vi "SerialASCII.vi"(11 "SerialASCIISettings":T1={"SerialPort"="RS232\\Port1", "TxFIFO"="DLRS1ADisplacementTxFIFO", "RxFIFO"="DLRS1ADisplacementRxFIFO", "TimestampRegister"="TimestampRegister", "Terminator"=10, "ReadTimeoutMs"=500}) -> ()   [LabVIEW 2016, in "FPGASerialASCII.lvlib"]
uses:
  FPGASerialASCII.lvlib
  DataTypes/SerialASCIISettings.ctl
  <vilib>/rvi/Emulation/niFpgaGetClockAttributes.vi
  <vilib>/rvi/Emulation/niFpgaSctlEmulationGetInTimedLoop.vi
  <vilib>/rvi/Emulation/niFpgaEmulationReportErrorSimple.vi
  <vilib>/rvi/DataTransferAndStorage/Container/Common/niFpgaContainerExecOnDevCompGetState.vi
  <vilib>/rvi/Emulation/niFpgaEmulationIsFPGAContextNoSignature.vi
  <vilib>/rvi/errors/niFpgaSetErrorForExecOnDevCompSimple.vi
  <vilib>/rvi/eio/common/nirviEmuReportErrorAndStop.vi
  <vilib>/rvi/DataTransferAndStorage/Container/Common/niFpgaContainerGetUniqueNameForEmu.vi
  <vilib>/rvi/FIFO/Fifo_Resource/nirvififoEmulationSetSize.vi
  <vilib>/rvi/FIFO/Fifo_Resource/nirviFifoEmulationQueueMgr.vi
  <instcachedir>/0/nirviFifoEmulationQueueMgr_E5CAEC123FF24DC58D834DCA3CDAA9B5.lvgen/nirviFifoEmulationQueueMgr_E5CAEC123FF24DC58D834DCA3CDAA9B5_009.vi
  <vilib>/rvi/FIFO/Fifo_Resource/nirvififoEmulationDetermineInputValidOut.vi
  <vilib>/rvi/FIFO/Fifo_Resource/nirvififoEmulationCreateLock.vi
  <vilib>/rvi/Emulation/niFpgaProcessEmulError.vi
  <vilib>/rvi/FIFO/Fifo_Resource/nirvififoEmulationObtainLock.vi
  <vilib>/rvi/FIFO/Fifo_Resource/nirvififoEmulationReleaseLock.vi
  <vilib>/rvi/occurrence/nirviWaitOnOccurrenceBase.vi
  <vilib>/rvi/errors/nirviReportUnexpectedCaseInternalError.vi
  <vilib>/rvi/errors/nirviReportUnexpectedCaseInternalError (U32).vi
  <vilib>/Utility/error.llb/Clear Errors.vi
  <vilib>/rvi/interface/RandomDataEmulation/niFpgaRandomDataHandleErrors.vi
  <vilib>/rvi/eio/common/nirviEmuTemplateMethod_errors.vi
  <vilib>/rvi/Memory/Memory_Emulation/niFpgaMemoryEmulationCacheClearOnFirstRun.vi
  <vilib>/rvi/Memory/Memory_Emulation/nirvimemoryEmulationManagerCache_MakeExclusive.vi
  <vilib>/rvi/Memory/Memory_Emulation/niFpgaMemoryEmulationValidateCache.vi
  <vilib>/rvi/Memory/Memory_Emulation/nirvimemoryEmulationManagerCache_InsertValue.vi
  <vilib>/rvi/Memory/Memory_Emulation/nirvimemoryEmulationManagerCache_ReleaseExclusive.vi
  <vilib>/rvi/Memory/Memory_Emulation/nirvimemoryEmulationManagerCache_GetValue.vi
  <vilib>/rvi/Memory/Memory_Emulation/nirvimemoryEmulationManagerCache_SetValue.vi
  <vilib>/rvi/Emulation/niFpgaCriticalErrorInLSC.vi
  <vilib>/rvi/DataTransferAndStorage/Container/XNode/niFpgaContainer.xnode
  <vilib>/rvi/FIFO/Fifo_Resource/niFpgaFifoEmulationRefIn.vi
  <vilib>/eio/EIOMethodNode/EIOMethodNode.xnode
  <vilib>/rvi/DataTransferAndStorage/Register/Emulation/niFpgaRegisterEmulationRefIn.vi
  Common_FPGA_FIFO/FPGAFIFO.lvlib
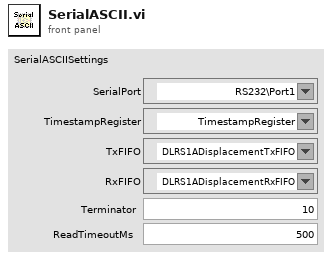
[diagram p1: front panel]
types:
  T1 = typedef "FPGASerialASCII.lvlib/SerialASCIISettings.ctl" = cluster{"SerialPort":refnum<k21>, "TxFIFO":refnum<k21>, "RxFIFO":refnum<k21>, "TimestampRegister":refnum<k21>, "Terminator":u8, "ReadTimeoutMs":i16}
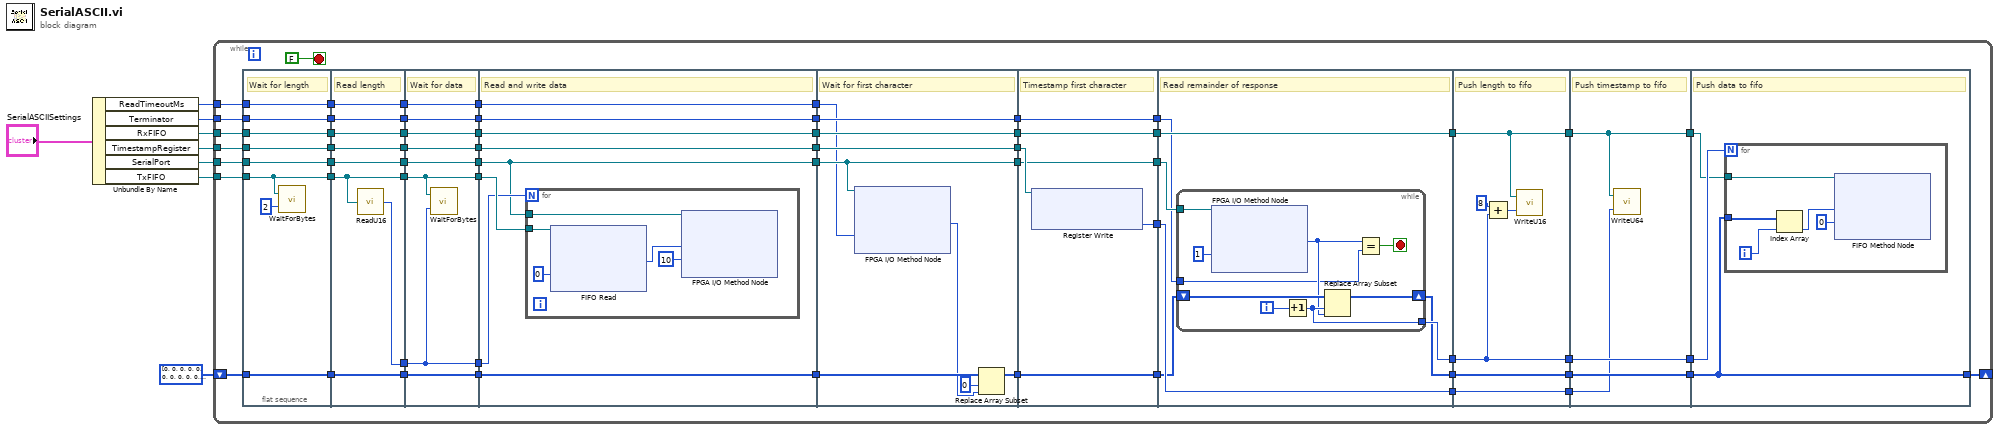
[diagram p0: block diagram]
diagram:
  n1 = Unbundle By Name("SerialASCIISettings") -> ("ReadTimeoutMs"=w1:i16, "Terminator"=w4:u8, "RxFIFO"=w6:refnum<k21>, "TimestampRegister"=w8:refnum<k21>, "SerialPort"=w2:refnum<k21>, "TxFIFO"=w5:refnum<k21>)
  n2 = while {
    tunnel: w2 -> [w67]
    tunnel: w8 -> [w66]
    shift-right: [w59] -> _
    shift-left: u8[] [0, 0, 0, 0, 0, 0, 0, 0, 0, 0, 0, 0, 0, 0, 0, 0, 0, 0, 0, 0, 0, 0, 0, 0, 0, 0, 0, 0, 0, 0, 0, 0, 0, 0, 0, 0, 0, 0, 0, 0, 0, 0, 0, 0, 0, 0, 0, 0, 0, 0, 0, 0, 0, 0, 0, 0, 0, 0, 0, 0, 0, 0, 0, 0, 0, 0, 0, 0, 0, 0, 0, 0, 0, 0, 0, 0, 0, 0, 0, 0, 0, 0, 0, 0, 0, 0, 0, 0, 0, 0, 0, 0, 0, 0, 0, 0, 0, 0, 0, 0, 0, 0, 0, 0, 0, 0, 0, 0, 0, 0, 0, 0, 0, 0, 0, 0, 0, 0, 0, 0, 0, 0, 0, 0, 0, 0, 0, 0, 0, 0, 0, 0, 0, 0, 0, 0, 0, 0, 0, 0, 0, 0, 0, 0, 0, 0, 0, 0, 0, 0, 0, 0, 0, 0, 0, 0, 0, 0, 0, 0, 0, 0, 0, 0, 0, 0, 0, 0, 0, 0, 0, 0, 0, 0, 0, 0, 0, 0, 0, 0, 0, 0, 0, 0, 0, 0, 0, 0, 0, 0, 0, 0, 0, 0, 0, 0, 0, 0, 0, 0, 0, 0, 0, 0, 0, 0, 0, 0, 0, 0, 0, 0, 0, 0, 0, 0, 0, 0, 0, 0, 0, 0, 0, 0, 0, 0, 0, 0, 0, 0, 0, 0, 0, 0, 0, 0, 0, 0, 0, 0, 0, 0, 0, 0, 0, 0, 0, 0, 0, 0, 0, 0, 0, 0, 0, 0] -> [w63]
    tunnel: w6 -> [w61]
    tunnel: w5 -> [w51]
    tunnel: w4 -> [w20]
    tunnel: w1 -> [w9]
    stop <- FALSE stop-if-true
    n3 = flat-sequence {
      tunnel: w51 -> [w70]
      tunnel: w61 -> [w72]
      tunnel: w63 -> [w73]
      tunnel: w66 -> [w74]
      tunnel: w67 -> [w75]
      tunnel: [w75] -> w50
      tunnel: [w74] -> w49
      tunnel: [w73] -> w48
      tunnel: [w72] -> w47
      tunnel: [w70] -> w46
      tunnel: w20 -> [w69]
      tunnel: [w69] -> w18
      tunnel: [w68] -> w10
      tunnel: w9 -> [w68]
      tunnel: w50 -> [w83]
      tunnel: [w83] -> w45
      tunnel: w49 -> [w82]
      tunnel: [w82] -> w43
      tunnel: w48 -> [w81]
      tunnel: [w81] -> w41
      tunnel: w47 -> [w80]
      tunnel: [w80] -> w39
      tunnel: w46 -> [w79]
      tunnel: [w79] -> w37
      tunnel: [w78] -> w35
      tunnel: [w77] -> w19
      tunnel: w18 -> [w77]
      tunnel: [w76] -> w11
      tunnel: w10 -> [w76]
      tunnel: w45 -> [w91]
      tunnel: [w91] -> w44
      tunnel: w43 -> [w90]
      tunnel: [w90] -> w42
      tunnel: w41 -> [w89]
      tunnel: [w89] -> w40
      tunnel: w39 -> [w88]
      tunnel: [w88] -> w38
      tunnel: w37 -> [w86]
      tunnel: [w86] -> w36
      tunnel: w35 -> [w87]
      tunnel: [w87] -> w34
      tunnel: w19 -> [w85]
      tunnel: [w85] -> w16
      tunnel: [w84] -> w12
      tunnel: w11 -> [w84]
      tunnel: [w95] -> w33
      tunnel: [w99] -> w31
      tunnel: [w98] -> w28
      tunnel: w44 -> [w95]
      tunnel: w42 -> [w99]
      tunnel: w40 -> [w94]
      tunnel: w38 -> [w98]
      tunnel: w36 -> [w97]
      tunnel: w34 -> [w96]
      tunnel: [w94] -> w26
      tunnel: [w93] -> w17
      tunnel: w16 -> [w93]
      tunnel: [w92] -> w13
      tunnel: w12 -> [w92]
      tunnel: w33 -> [w107]
      tunnel: [w107] -> w32
      tunnel: w31 -> [w113]
      tunnel: [w113] -> w30
      tunnel: [w109] -> w29
      tunnel: w28 -> [w112]
      tunnel: [w112] -> w27
      tunnel: w26 -> [w110]
      tunnel: w17 -> [w106]
      tunnel: [w106] -> w14
      tunnel: w13 -> [w105]
      tunnel: w32 -> [w117]
      tunnel: w30 -> [w119]
      tunnel: [w118] -> w65
      tunnel: [w117] -> w64
      tunnel: w29 -> [w116]
      tunnel: [w116] -> w62
      tunnel: w27 -> [w115]
      tunnel: [w115] -> w60
      tunnel: [w114] -> w15
      tunnel: w14 -> [w114]
      tunnel: w65 -> [w123]
      tunnel: w64 -> [w126]
      tunnel: w62 -> [w122]
      tunnel: [w125] -> w57
      tunnel: w60 -> [w124]
      tunnel: [w124] -> w56
      tunnel: [w123] -> w25
      tunnel: [w121] -> w23
      tunnel: w15 -> [w120]
      tunnel: w57 -> [w141]
      tunnel: [w141] -> w55
      tunnel: w56 -> [w137]
      tunnel: [w137] -> w53
      tunnel: w25 -> [w138]
      tunnel: [w139] -> w24
      tunnel: w23 -> [w139]
      tunnel: [w138] -> w21
      tunnel: w55 -> [w145]
      tunnel: [w145] -> w54
      tunnel: w53 -> [w143]
      tunnel: [w143] -> w52
      tunnel: w24 -> [w144]
      tunnel: [w144] -> w22
      tunnel: w21 -> [w142]
      tunnel: w54 -> [w148]
      tunnel: w52 -> [w147]
      tunnel: [w146] -> w59
      tunnel: w22 -> [w146]
      frame #0 {
        # "Wait for length"
        n4 = call "WaitForBytes.vi"("Bytes"=u16 2, "FIFO"=w70) -> ()  [unwired: 1 in]
      }
      frame #1 {
        # "Read length"
        n5 = call "ReadU16.vi"("FIFO"=w79) -> ("U16"=w78:u16)
      }
      frame #2 {
        # "Wait for data"
        n6 = call "WaitForBytes.vi"("Bytes"=w87, "FIFO"=w86) -> ()  [unwired: 1 in]
      }
      frame #3 {
        # "Read and write data"
        n7 = for {
          N: w96 -> [_]
          tunnel: w97 -> [w104]
          tunnel: w95 -> [w102]
          n8 = xnode "FIFO Read"("Timeout"=0, "FIFO In"=w104) -> ("Element"=w101:u8)  [unwired: 2 out]
          n9 = xnode "FPGA I/O Method Node"("FPGA I/O In"=w102, "Data"=w101, "Timeout (ms)"=10) -> ()  [unwired: 2 out]
        }
      }
      frame #4 {
        # "Wait for first character"
        n10 = xnode "FPGA I/O Method Node"("FPGA I/O In"=w107, "Timeout (ms)"=w105) -> ("Data"=w108:u8)  [unwired: 2 out]
        n11 = Replace Array Subset(array=w110, new element=w108, index=0) -> (w109:u8[])
      }
      frame #5 {
        # "Timestamp first character"
        n12 = xnode "Register Write"("Register In"=w119) -> ("Data"=w118:u64)  [unwired: 1 out]
      }
      frame #6 {
        # "Read remainder of response"
        n13 = while {
          tunnel: w126 -> [w135]
          shift-right: [w131] -> w121
          shift-left: w122 -> [w133]
          tunnel: [w130] -> w125
          tunnel: w120 -> [w127]
          i -> [w132]
          stop <- w134 stop-if-true
          n14 = xnode "FPGA I/O Method Node"("FPGA I/O In"=w135, "Timeout (ms)"=1) -> ("Data"=w129:u8)  [unwired: 2 out]
          n15 = Increment(x=w132) -> (x+1=w130:i32)
          n16 = Replace Array Subset(array=w133, new element=w129, index=w130) -> (w131:u8[])
          n17 = Equal?(x=w129, y=w127) -> (x = y?=w134:bool)
        }
      }
      frame #7 {
        # "Push length to fifo"
        n18 = Add(x=8, y=w141) -> (x+y=w136:i32)
        n19 = call "WriteU16.vi"("U16"=w136, "FIFO"=w137) -> ()  [unwired: 1 in]
      }
      frame #8 {
        # "Push timestamp to fifo"
        n20 = call "WriteU64.vi"("U64"=w142, "FIFO"=w143) -> ()  [unwired: 1 in]
      }
      frame #9 {
        # "Push data to fifo"
        n21 = for {
          N: w148 -> [_]
          tunnel: w146 -> [w153]
          tunnel: w147 -> [w152]
          i -> [w150]
          n22 = Index Array(array=w153, index=w150) -> (element=w151:u8)
          n23 = xnode ("FIFO Method Node")("Element"=w151, "Timeout"=0, "FIFO In"=w152) -> ()  [unwired: 2 out]
        }
      }
    }
  }
